vi "Append PDF file to PDF Report .vi"(0 "PDF Report":refnum<class "PDF Report Class.lvclass">, 7 "PDF Files  to concatenate and pages":T1={"Path"=path "", "Pages"="all", "Password"=""}, 11 "error in (no error)":errorcluster) -> (4 "PDF Report duplicate":refnum<class "PDF Report Class.lvclass">, 15 "error out":errorcluster)   [LabVIEW 2019]
doc: "We use PDF Copy to import a page: All interactive features (annotations, bookmarks, fields, and so forth) of the imported page are still there. A page is imported with his exact dimensions.\n\nVersion 1.0\nDeveloped by Jean-Marc Simard\nCopyright © 2012, Exaprom Inc.\nAll rights reserved.\nLicense: BSD\n\nWith iTextSharp Library\n(http://itextsharp.sourceforge.net)"
uses:
  <userlib>/Exaprom PDF/LV Class/PDF Report Class/PDF Report Class.lvclass
  <userlib>/Exaprom PDF/Controls/Concatenate Controls/PDF file to concatenate.ctl
  <userlib>/Exaprom PDF/Controls/Concatenate Controls/PDF File and position.ctl
  <userlib>/Exaprom PDF/Controls/Concatenate Controls/PDF file source.ctl
  C:/Program Files/National Instruments/LabVIEW 2019/user.lib/Exaprom PDF/DLL/itextsharp.dll
  DLL/itextsharp.dll
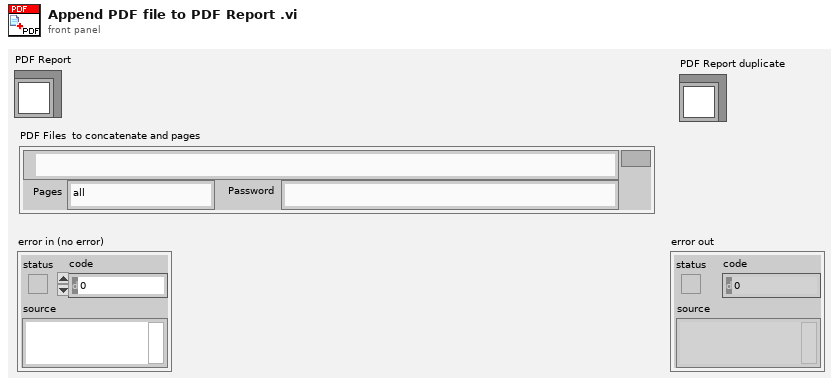
[diagram p1: front panel]
types:
  T1 = typedef "PDF file to concatenate.ctl" = cluster{"Path":path, "Pages":string, "Password":string}
  T2 = typedef "PDF File and position.ctl" = cluster{"Path":path, "Pages":string, "Source":T3, "Start at page old":i32, "Start at page new":i32, "Owner password":string}
  T3 = typedef "PDF file source.ctl" = enum16{"PDF Report", "File to add"}
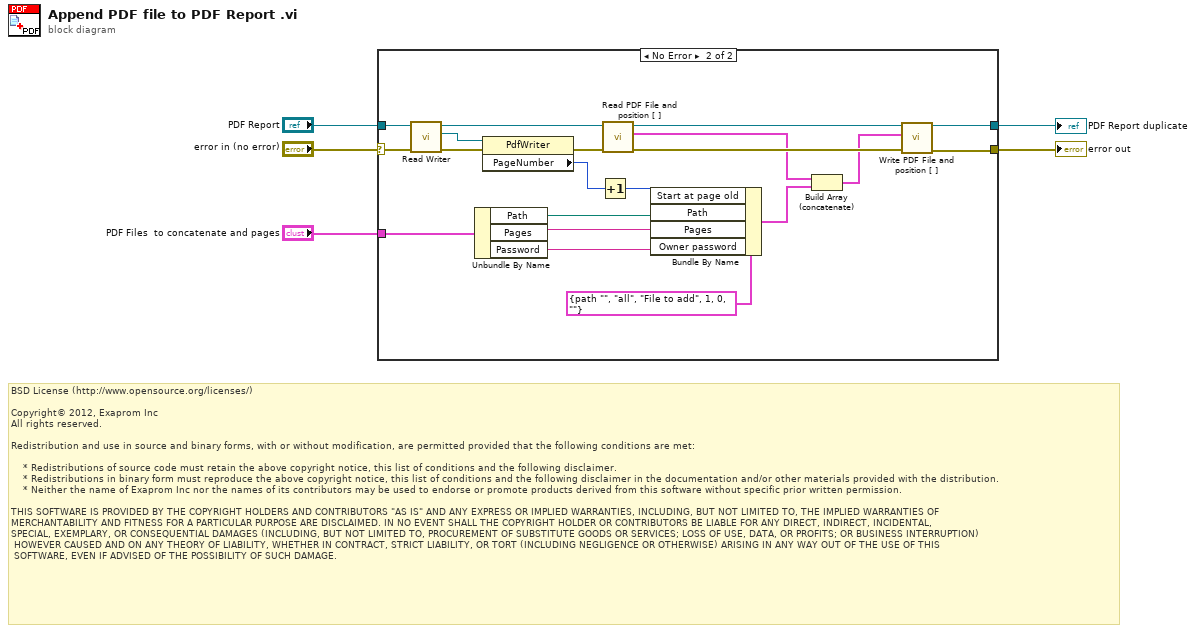
[diagram p0: block diagram]
diagram:
  # "BSD License (http://www.opensource.org/licenses/)\n\nCopyright© 2012, Exaprom Inc\nAll rights reserved.\n\nRedistribution and use in source and binary forms, with or without modification, are permitted provided that the following conditions are met:\n\n    * Redistributions of source code must retain the above copyright notice, this list of conditions and the following disclaimer.\n    * Redistributions in binary form must reproduce the above copyright notice, this list of conditions and the following disclaimer in the documentation and/or other materials provided with the distribution.\n    * Neither the name of Exaprom Inc nor the names of its contributors may be used to endorse or promote products derived from this software without specific prior written permission.\n\nTHIS SOFTWARE IS PROVIDED BY THE COPYRIGHT HOLDERS AND CONTRIBUTORS \"AS IS\" AND ANY EXPRESS OR IMPLIED WARRANTIES, INCLUDING, BUT NOT LIMITED TO, THE IMPLIED WARRANTIES OF \nMERCHANTABILITY AND FITNESS FOR A PARTICULAR PURPOSE ARE DISCLAIMED. IN NO EVENT SHALL THE COPYRIGHT HOLDER OR CONTRIBUTORS BE LIABLE FOR ANY DIRECT, INDIRECT, INCIDENTAL,\nSPECIAL, EXEMPLARY, OR CONSEQUENTIAL DAMAGES (INCLUDING, BUT NOT LIMITED TO, PROCUREMENT OF SUBSTITUTE GOODS OR SERVICES; LOSS OF USE, DATA, OR PROFITS; OR BUSINESS INTERRUPTION)\n HOWEVER CAUSED AND ON ANY THEORY OF LIABILITY, WHETHER IN CONTRACT, STRICT LIABILITY, OR TORT (INCLUDING NEGLIGENCE OR OTHERWISE) ARISING IN ANY WAY OUT OF THE USE OF THIS\n SOFTWARE, EVEN IF ADVISED OF THE POSSIBILITY OF SUCH DAMAGE."
  n1 = case shown="No Error" "error in (no error)" {
    selector: "error in (no error)" -> [w7 w23]
    tunnel: [w7 w26] -> w5
    tunnel: "PDF Report" -> [w6 w27]
    tunnel: [w6 w25] -> w2
    tunnel: "PDF Files  to concatenate and pages" -> [_ w24]
    frame Error {
    }
    frame No Error {
      n2 = call-dynamic "Read Writer.vi"("error in (no error)"=w23, "PDF Report Class in"=w27) -> ("error out"=w21:errorcluster, "Writer"=w20:refnum<k24>, "PDF Report Class out"=w22:refnum<class "PDF Report Class.lvclass">)  [unwired: 7 in]
      n3 = Unbundle By Name(w24) -> ("Path"=w17:path, "Pages"=w16:string, "Password"=w8:string)
      n4 = property class="PdfWriter"(reference=w20, error in=w21) -> (error out=w19:errorcluster, "PageNumber"=w10:i32)  [unwired: 1 out]
      n5 = Increment(x=w10) -> (x+1=w9:i32)
      n6 = call-dynamic "Read PDF File and position [ ].vi"("error in (no error)"=w19, "PDF Report Class in"=w22) -> ("error out"=w14:errorcluster, "PDF File and position [ ]"=w13:T2[], "PDF Report Class out"=w15:refnum<class "PDF Report Class.lvclass">)  [unwired: 7 in]
      n7 = Bundle By Name(cluster=T2 {"Path"=path "", "Pages"="all", "Source"=enum."File to add", "Start at page old"=1, "Start at page new"=0, "Owner password"=""} ("PDF File and position"), "Start at page old"=w9, "Path"=w17, "Pages"=w16, "Owner password"=w8) -> (w12:T2)
      n8 = Build Array (concatenate)(w13, w12) -> (w11:T2[])
      n9 = call-dynamic "Write PDF File and position [ ].vi"("error in (no error)"=w14, "PDF File and position [ ]"=w11, "PDF Report Class in"=w15) -> ("error out"=w26:errorcluster, "PDF Report Class out"=w25:refnum<class "PDF Report Class.lvclass">)  [unwired: 7 in]
    }
  }
  "error out" <- w5
  "PDF Report duplicate" <- w2
